vi "UniqueLast_I.vi"(11 "1D Array In":i32[](array[numeric])) -> (3 "Boolean":bool)   [LabVIEW 2009]
uses:
  ArrayLast_I.vi
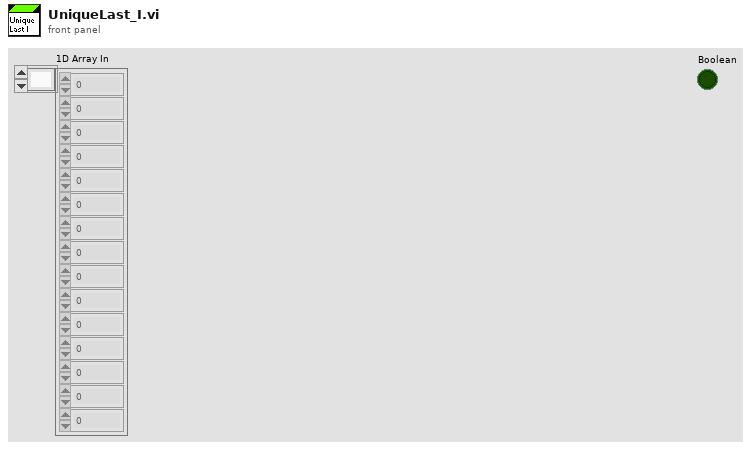
[diagram p1: front panel]
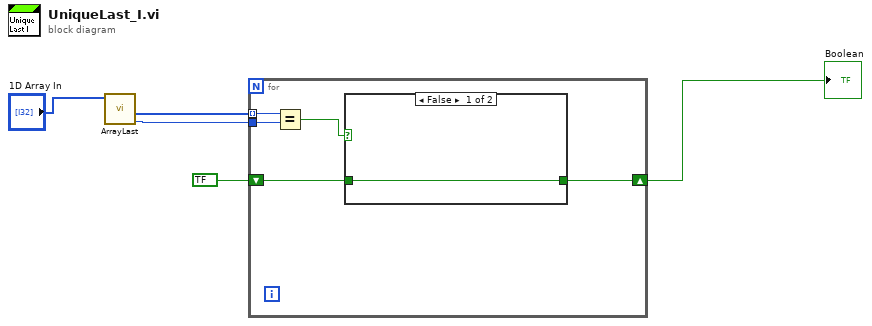
[diagram p0: block diagram]
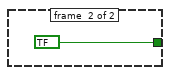
[diagram p2: hidden frame]
diagram:
  n1 = call-poly "ArrayLast.vi"("1D Array In"="1D Array In") -> ("Last Element"=w2:i32, "Head of Array"=w3:i32[])  [unwired: 9 in]
  n2 = for {
    shift-right: [w7] -> w1
    shift-left: bool ? -> [w6]
    tunnel: w3 -> [w10] mode=indexing
    tunnel: w2 -> [w9]
    n3 = Equal?(x=w10, y=w9) -> (x = y?=w8:bool)
    n4 = case shown="False" w8 {
      tunnel: [w11 bool ?] -> w7
      tunnel: w6 -> [w11 _]
      frame #0 {
      }
      frame #1 {
      }
    }
  }
  "Boolean" <- w1
